vi "Insert Above.vi"(8 "error in (no error)":errorcluster, 9 "Item Tag":string, 10 "Tree Refnum":refnum<vi>, 11 "Tree Click Interpreter in":refnum<class "Tree Click Interpreter.lvclass">) -> (0 "error out":errorcluster, 1 "Insertion Index":i32, 2 "Parent ID":string, 3 "Tree Click Interpreter out":refnum<class "Tree Click Interpreter.lvclass">)   [LabVIEW 2017, in "Tree Click Interpreter.lvclass"]
uses:
  Tree Click Interpreter.lvclass
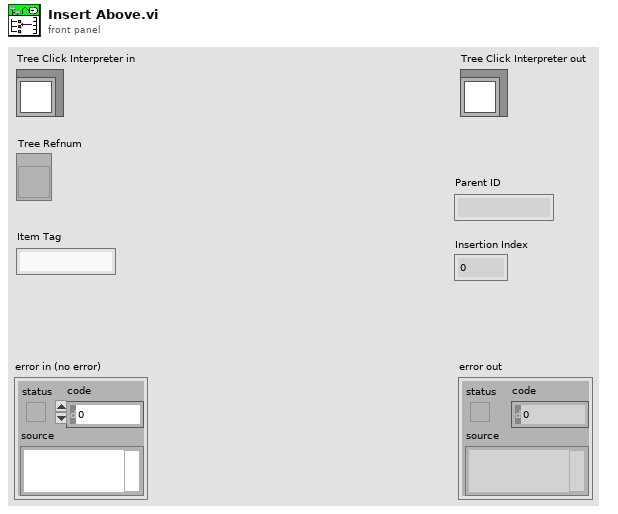
[diagram p1: front panel]
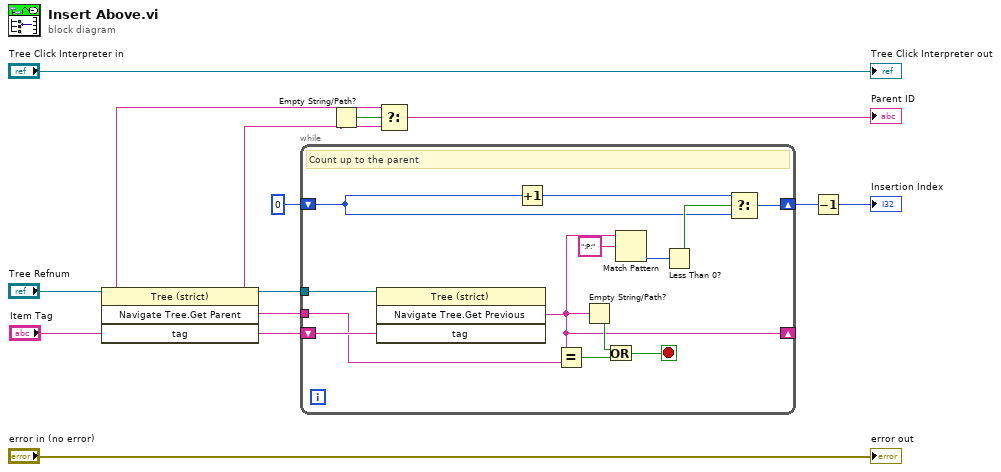
[diagram p0: block diagram]
diagram:
  n1 = invoke class="Tree (strict)" method="Navigate Tree.Get Parent"(reference="Tree Refnum", "tag"="Item Tag") -> (reference out=w8:refnum<vi>, "Navigate Tree:Get Parent"=w6:string)  [unwired: 2 in, 2 out]
  n2 = while {
    shift-right: [w12] -> w2
    shift-left: 0 -> [w14]
    tunnel: w8 -> [w24]
    tunnel: w6 -> [w22]
    shift-right: [w18] -> _
    shift-left: "Item Tag" -> [w23]
    stop <- w19 stop-if-true
    # "Count up to the parent"
    n3 = invoke class="Tree (strict)" method="Navigate Tree.Get Previous"(reference=w24, "tag"=w23) -> ("Navigate Tree:Get Previous"=w18:string)  [unwired: 2 in, 3 out]
    n4 = Increment(x=w14) -> (x+1=w13:i32)
    n5 = Equal?(x=w18, y=w22) -> (x = y?=w21:bool)
    n6 = Empty String/Path?(string/path=w18) -> (empty?=w20:bool)
    n7 = Or(x=w20, y=w21) -> (x .or. y?=w19:bool)
    n8 = Match Pattern(string=w18, regular expression=":P:") -> (offset past match=w16:i32)  [unwired: 1 in, 3 out]
    n9 = Less Than 0?(x=w16) -> (x < 0?=w15:bool)
    n10 = Select(t=w13, s=w15, f=w14) -> (s? t:f=w12:i32)
  }
  n11 = Empty String/Path?(string/path=w6) -> (empty?=w7:bool)
  n12 = Select(t="Item Tag", s=w7, f=w6) -> (s? t:f=→"Parent ID":string)
  n13 = Decrement(x=w2) -> (x-1=→"Insertion Index":i32)
  "error out" <- "error in (no error)"
  "Tree Click Interpreter out" <- "Tree Click Interpreter in"
